vi "Set Results.vi"(8 "error in (no error)":errorcluster, 10 "Sequence Context":refnum<k7>, 11 "PostUUT in":refnum<class "PostUUT.lvclass">) -> (0 "error out":errorcluster, 3 "PostUUT out":refnum<class "PostUUT.lvclass">)   [LabVIEW 2019, in "OPC UA.lvlib" / "PostUUT.lvclass"]
uses:
  PostUUT.lvclass
  C:/Workspace/BSM OOP/Sequence/CodeModules/OPC UA Client/OPC UA/OPC UA.lvclass
  OPC UA/OPC UA.lvclass/OPC UA.ctl
  <vilib>/addons/TestStand/_TSUtility.llb/TestStand - Get Property Value (Number {Signed 32-bit Integer}).vi
  <vilib>/addons/TestStand/_TSUtility.llb/TestStand - Get Property Value (String).vi
  <vilib>/addons/TestStand/_TSUtility.llb/TestStand - Set Property Value (Boolean).vi
  OPC UA/OPC UA.lvclass
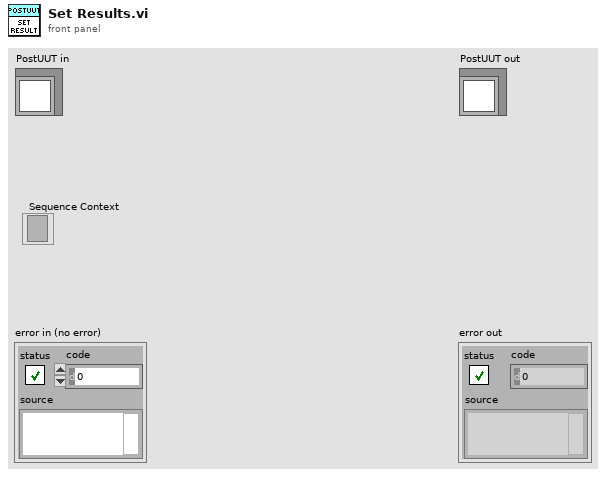
[diagram p1: front panel]
types:
  T1 = cluster{"Result":i32, "Result Status":string, "Elapsed Time":i32}
  T2 = typedef "LVDateTimeRec.ctl" = cluster{"fractional second":dbl, "second":i32, "minute":i32, "hour":i32, "day of month":i32, "month":i32, "year":i32, "day of week":i32, "day of year":i32, "DST":i32}
  T3 = cluster{"fractional second":i32, "second":i32, "minute":i32, "hour":i32, "day of month":i32, "month":i32, "year":i32, "day of week":i32, "day of year":i32, "DST":i32}
  T4 = typedef "OPC UA.lvlib/OPC UA.lvclass/Tester Tx Dataset.ctl" = cluster{"Fault":bool, "StepNo":u32, "Ready":bool, "HighVoltage":bool, "TestRunning":bool, "ResultsReady":bool, "Results":u32, "ElapsedTime":u32, "Online":bool, "TimeCompleted":i32[], "Timeout":bool, "Heartbeat":bool}
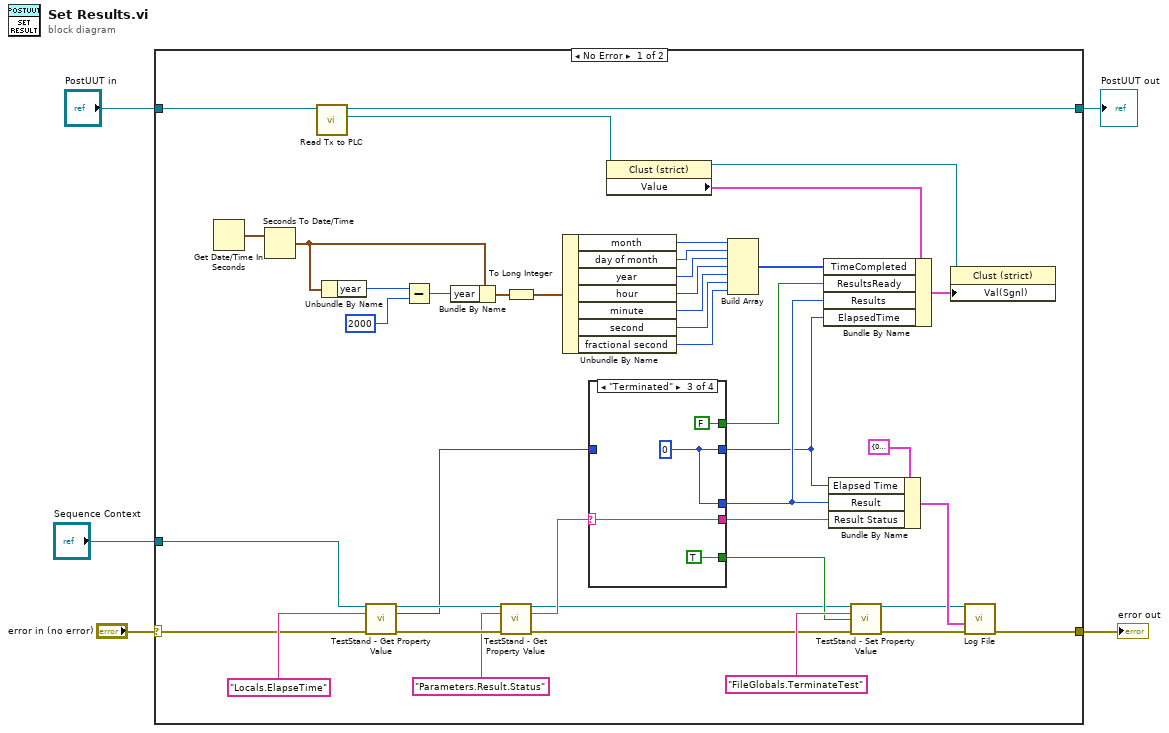
[diagram p0: block diagram]
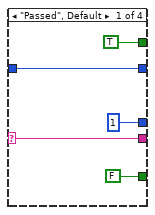
[diagram p2: hidden frame]
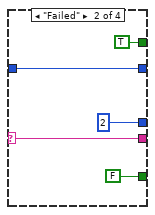
[diagram p3: hidden frame]
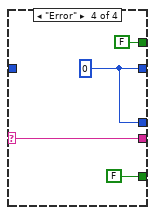
[diagram p4: hidden frame]
diagram:
  n1 = case shown="No Error" "error in (no error)" {
    selector: "error in (no error)" -> [w13 w67]
    tunnel: [w15 w67] -> w4
    tunnel: [w9 w66] -> w2
    tunnel: "PostUUT in" -> [w7 w66]
    tunnel: "Sequence Context" -> [w6 _]
    frame No Error {
      n2 = Get Date/Time In Seconds() -> (seconds since 1Jan1904=w46:timestamp)
      n3 = Seconds To Date/Time(time stamp (now)=w46) -> (date time rec=w35:T2)  [unwired: 1 in]
      n4 = call "Read Tx to PLC.vi"("OPC UA in"=w7) -> ("Tx to PLC"=w8:refnum<vi>, "OPC UA out"=w9:refnum<class "PostUUT.lvclass">)  [unwired: 8 in, 1 out]
      n5 = Unbundle By Name(w35) -> ("year"=w33:i32)
      n6 = call-poly <vilib>:"TestStand - Get Property Value.vi"("Sequence Context In"=w6, "Lookup String"="Locals.ElapseTime", "error in (no error)"=w13) -> ("Sequence Context Out"=w27:refnum<k7>, "Value"=w11:i32, "error out"=w30:errorcluster)  [unwired: 10 in]
      n7 = Subtract(x=w33, y=2000) -> (x-y=w36:i32)
      n8 = Bundle By Name(cluster=w35, "year"=w36) -> (w37:T2)
      n9 = call-poly <vilib>:"TestStand - Get Property Value.vi"("Sequence Context In"=w27, "Lookup String"="Parameters.Result.Status", "error in (no error)"=w30) -> ("Sequence Context Out"=w22:refnum<k7>, "Value"=w26:string, "error out"=w24:errorcluster)  [unwired: 10 in]
      n10 = To Long Integer(number=w37) -> (32bit integer=w38:T3)
      n11 = Unbundle By Name(w38) -> ("month"=w39:i32, "day of month"=w40:i32, "year"=w41:i32, "hour"=w42:i32, "minute"=w43:i32, "second"=w44:i32, "fractional second"=w45:i32)
      n12 = case shown="\"Terminated\"" w26 {
        selector: w26 -> [w51 w56 w61 w65]
        tunnel: [1 2 w58 w62] -> w20
        tunnel: [w51 w56 w61 w65] -> w19
        tunnel: [FALSE ("ResultsReady") FALSE ("ResultsReady") TRUE ("ResultsReady") FALSE ("ResultsReady")] -> w23
        tunnel: [TRUE ("ResultsReady") TRUE ("ResultsReady") FALSE ("ResultsReady") FALSE ("ResultsReady")] -> w12
        tunnel: w11 -> [w48 w53 _ _]
        tunnel: [w48 w53 w58 w62] -> w10
        frame "Passed", Default {
        }
        frame "Failed" {
        }
        frame "Terminated" {
          w58 = 0 ("Value")
        }
        frame "Error" {
          w62 = 0 ("Value")
        }
      }
      n13 = property class="Clust (strict)"(reference=w8) -> (reference out=w31:refnum<vi>, "Value"=w32:T4)  [unwired: 1 in, 1 out]
      n14 = Build Array(w39, w40, w41, w42, w43, w44, w45) -> (w47:i32[])
      n15 = Bundle By Name(cluster=w32, "TimeCompleted"=w47, "ResultsReady"=w12, "Results"=w20, "ElapsedTime"=w10) -> (w14:T4)
      n16 = Bundle By Name(cluster=T1 {"Result"=0, "Result Status"="", "Elapsed Time"=0}, "Elapsed Time"=w10, "Result"=w20, "Result Status"=w19) -> (w17:T1)
      n17 = call-poly <vilib>:"TestStand - Set Property Value.vi"("Sequence Context In"=w22, "Lookup String"="FileGlobals.TerminateTest", "New Value"=w23, "error in (no error)"=w24) -> ("Sequence Context Out"=w16:refnum<k7>, "error out"=w18:errorcluster)  [unwired: 10 in]
      n18 = property class="Clust (strict)"(reference=w31, "Val(Sgnl)"=w14) -> ()  [unwired: 1 in, 2 out]
      n19 = call "Log File.vi"("error in"=w18, "Test Result"=w17, "Sequence Context"=w16) -> ("error out"=w15:errorcluster)  [unwired: 8 in]
    }
    frame Error {
    }
  }
  "error out" <- w4
  "PostUUT out" <- w2
